vi "Init-FileHandler.vi"(6 "Flush Timeout (5 s)":dbl=5.0, 7 "Filepath":path, 8 "error in":errorcluster, 9 "Level":T1, 10 "Name":string, 11 "FileHandler":refnum<class "FileHandler.lvclass">) -> (0 "error out":errorcluster, 3 "FileHandler out":refnum<class "FileHandler.lvclass">)   [LabVIEW 2020, in "hse-logger.lvlib" / "FileHandler.lvclass"]
doc: "Initiates a new FileHandler-object with a name, log-level and a filepath for the log-file.\nThe handler processes LogRecords only if the level of the handler is greater or equal to the level of the LogRecord.\n\n____\nHAMPEL SOFTWARE ENGINEERING v2.0.6 (2021-04-15 11:38)"
uses:
  FileHandler.lvclass
  LogLevel.ctl
  FileHandler.lvclass/FileHandler.ctl
  hse-logger.lvlib
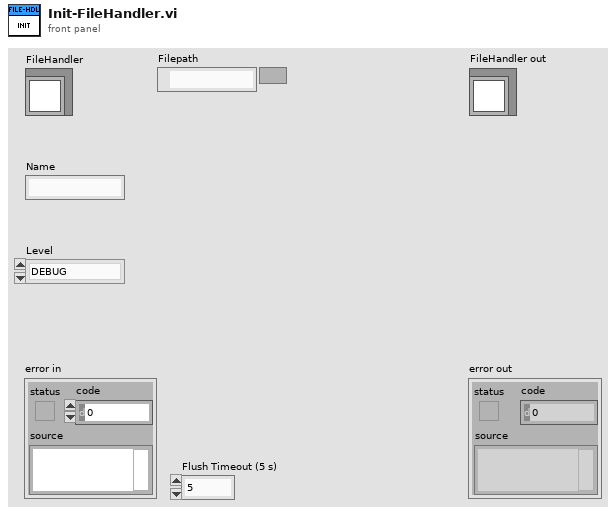
[diagram p1: front panel]
types:
  T1 = typedef "hse-logger.lvlib/LogLevel.ctl" = enum16{"DEBUG", "INFO", "WARNING", "ERROR", "CRITICAL"}
  T2 = enum16{"open", "replace", "create", "open or create", "replace or create", "replace or create with confirmation"}
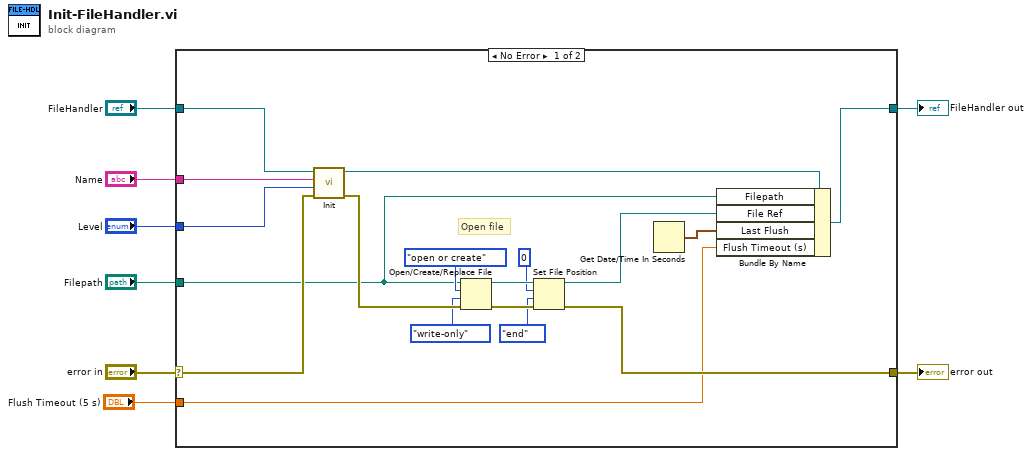
[diagram p0: block diagram]
diagram:
  n1 = case shown="No Error" "error in" {
    selector: "error in" -> [w25 w28]
    tunnel: [w16 w28] -> w7
    tunnel: [w24 w27] -> w6
    tunnel: "Name" -> [w15 _]
    tunnel: "Level" -> [w14 _]
    tunnel: "Filepath" -> [w17 _]
    tunnel: "FileHandler" -> [w13 w27]
    tunnel: "Flush Timeout (5 s)" -> [w10 _]
    frame No Error {
      # "Open file"
      n2 = call-dynamic "Init.vi"("error in"=w25, "Level"=w14, "Name"=w15, "Handler"=w13) -> ("error out"=w26:errorcluster, "Handler out"=w12:refnum<class "FileHandler.lvclass">)  [unwired: 6 in]
      n3 = Open/Create/Replace File(file path (use dialog)=w17, error in=w26, operation (0:open)=T2."open or create", access (0:read/write)=enum16{"read/write", "read-only", "write-only"}."write-only") -> (refnum out=w21:refnum<file>, error out=w22:errorcluster)  [unwired: 2 in, 1 out]
      n4 = Set File Position(offset (in bytes) (0)=i64 0, refnum=w21, from (0:start)=enum16{"start", "end", "current"}."end", error in=w22) -> (refnum out=w11:refnum<file>, error out=w16:errorcluster)
      n5 = Get Date/Time In Seconds() -> (seconds since 1Jan1904=w9:timestamp)
      n6 = Bundle By Name(cluster=w12, "Filepath"=w17, "File Ref"=w11, "Last Flush"=w9, "Flush Timeout (s)"=w10) -> (w24:refnum<class "FileHandler.lvclass">)
    }
    frame Error {
    }
  }
  "error out" <- w7
  "FileHandler out" <- w6
